vi "Update Autocomplete Variables.vi"(11 "UI Data in":refnum<class "Settings UI.lvclass">) -> (3 "UI Data out":refnum<class "Settings UI.lvclass">)   [LabVIEW 2020, in "Output Sequencer.lvlib" / "Settings UI.lvclass"]
uses:
  Settings UI.lvclass
  Settings UI.lvclass/Settings UI.ctl
  Output Sequencer/Globals/Global Strings.vi
  Output Sequencer/Output Sequencer.lvclass
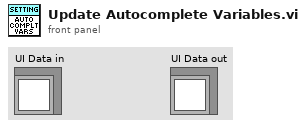
[diagram p1: front panel]
types:
  T1 = typedef "Output Sequencer.lvlib/Settings UI.lvclass/Tree Item Settings.ctl" = cluster{"Tree Label":string, "Indent Level":i32, "Data Type":T2, "Numeric Range":cluster{"Min":dbl, "Max":dbl, "Inc":dbl}, "Allowed Values":string[], "Default Value":string, "Description":string}
  T2 = typedef "Output Sequencer.lvlib/Settings UI.lvclass/Data Type.ctl" = i16
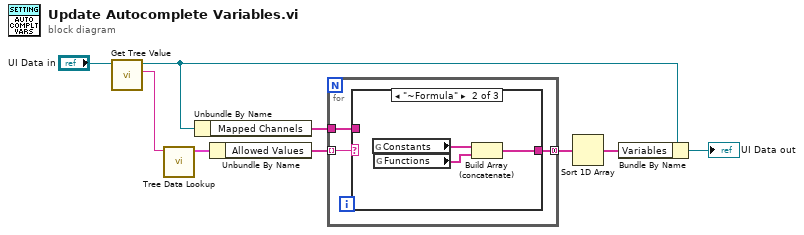
[diagram p0: block diagram]
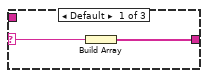
[diagram p2: hidden frame]
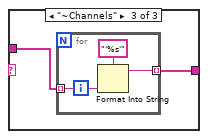
[diagram p3: hidden frame]
diagram:
  n1 = call "Get Tree Value.vi"("UI Data in"="UI Data in") -> ("Value"=w6:string, "UI Data out"=w4:refnum<class "Settings UI.lvclass">)  [unwired: 9 in]
  n2 = call "Tree Data Lookup.vi"("Tag in"=w6) -> ("Tree Data"=w7:T1)  [unwired: 5 in, 5 out]
  n3 = Unbundle By Name(w4) -> ("Mapped Channels"=w1:string[])
  n4 = Unbundle By Name(w7) -> ("Allowed Values"=w8:string[])
  n5 = for {
    tunnel: [w12] -> w3 mode=concatenating
    tunnel: w8 -> [w11] mode=indexing
    tunnel: w1 -> [w10]
    n6 = case shown="\"~Formula\"" w11 {
      selector: w11 -> [w14 _ _]
      tunnel: [w13 w15 w19] -> w12
      tunnel: w10 -> [_ _ w18]
      frame Default {
        n7 = Build Array(w14) -> (w13:string[])
      }
      frame "~Formula" {
        n8 = global read "Global Strings.vi" "Constants"() -> (w17:string[])
        n9 = global read "Global Strings.vi" "Functions"() -> (w16:string[])
        n10 = Build Array (concatenate)(w17, w16) -> (w15:string[])
      }
      frame "~Channels" {
        n11 = for {
          tunnel: [w22] -> w19 mode=indexing
          tunnel: w18 -> [w20] mode=indexing
          n12 = Format Into String(format string="'%s'", w20) -> (resulting string=w22:string)  [unwired: 2 in, 1 out]
        }
      }
    }
  }
  n13 = Sort 1D Array(array=w3) -> (sorted array=w2:string[])
  n14 = Bundle By Name(cluster=w4, "Variables"=w2) -> (→"UI Data out":refnum<class "Settings UI.lvclass">)
